vi "Poll iRobot and Accelerometer.vi"(6 "accel smoothing (0-1)":dbl=0.1, 8 "error in":errorcluster, 11 "UART port in":T10) -> (0 "error out":errorcluster, 1 "Acceleration (g)":T1 {"z axis (g)" format="%.3f"; "y axis (g)" format="%.3f"; "x axis (g)" format="%.3f"}, 2 "iRobot SensorGroup6":T2={"Bumps + Wheel Drops"={"Wheeldrop Caster"=FALSE, "Wheeldrop Left"=FALSE, "Wheeldrop Right"=FALSE, "Bump Left"=FALSE, "Bump Right"=FALSE}, "Wall"=FALSE, "Cliff Left"=FALSE, "Cliff Front Left"=FALSE, "Cliff Front Right"=FALSE, "Cliff Right"=FALSE, "Virtual Wall"=FALSE, "Low-Side Driver + Wheel Overcurrent"={"Low-Side Driver 0"=FALSE, "Low-Side Driver 1"=FALSE, "Low-Side Driver 2"=FALSE, "Left Wheel"=FALSE, "Right Wheel"=FALSE}, "Infrared"=255, "Buttons"={"Advance"=FALSE, "Play"=FALSE}, "Distance (mm)"=0, "Angle (deg)"=0, "Charging State"=enum."Not Charging", "Voltage (mV)"=0, "Current (mA)"=0, "Battery Temperature (deg C)"=0, "Battery Charge (mAh)"=0, "Battery Capacity (mAh)"=0, "Wall Signal (0-4095)"=0, "Cliff Left Signal (0-4095)"=0, "Cliff Front Left Signal (0-4095)"=0, "Cliff Front Right Signal (0-4095)"=0, "Cliff Right Signal (0-4095)"=0, "Cargo Bay Digital Inputs"={"Digital Input 0"=FALSE, "Digital Input 1"=FALSE, "Digital Input 2"=FALSE, "Digital Input 3"=FALSE, "Device Detect"=FALSE}, "Cargo Bay Analog Signal (0-1023)"=0, "Charging Sources Available"={"Internal Charger"=FALSE, "Home Base"=FALSE}, "OI Mode"=enum."Off", "Song Number"=0, "Song Playing"=FALSE, "Number of Stream Packets"=0, "Requested Velocity (mm/s)"=0, "Requested Radius (mm)"=0, "Requested Right Wheel Velocity (mm/s)"=0, "Requested Left Wheel Velocity (mm/s)"=0} {"Infrared" format="%02x"}, 3 "UART port out":T10, 5 "net angle (deg)":i32, 7 "net distance (mm)":i32)   [LabVIEW 2015]
uses:
  iRobot/Advanced/UART/iRobot UART Port Type.ctl
  iRobot/Sensor/Sensor Group 6.ctl
  iRobot/Sensor/Bumps + Wheel Drops.ctl
  iRobot/Sensor/Low-Side Driver + Wheel Overcurrent.ctl
  iRobot/Sensor/Buttons.ctl
  iRobot/Sensor/Charging State.ctl
  iRobot/Sensor/Cargo Bay Digital Inputs.ctl
  iRobot/Sensor/Charging Sources Available.ctl
  iRobot/Sensor/OI Mode.ctl
  Accelerometer.ctl
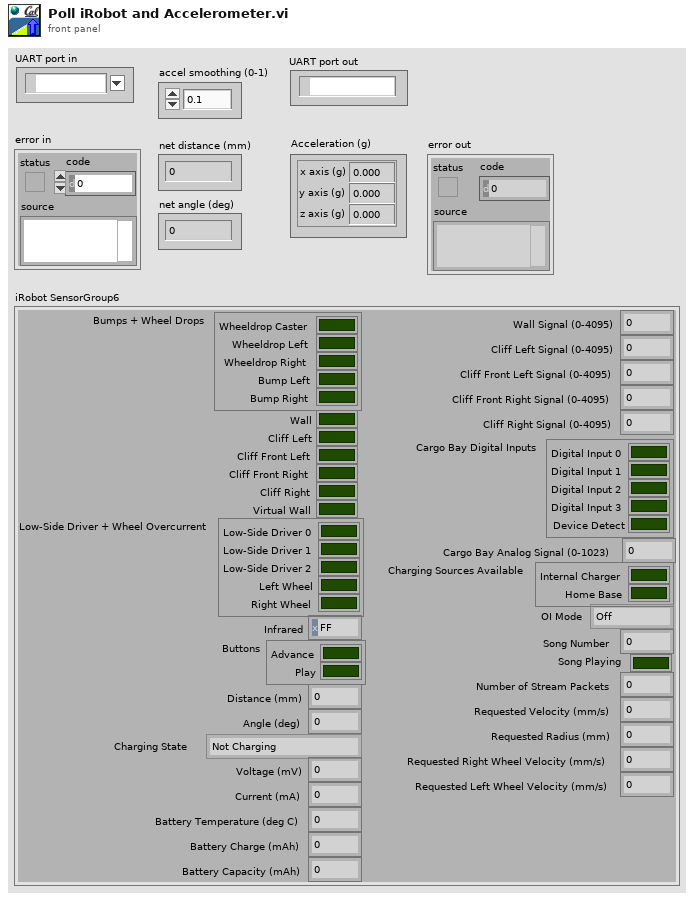
[diagram p1: front panel]
types:
  T1 = typedef "Accelerometer.ctl" = cluster{"x axis (g)":dbl, "y axis (g)":dbl, "z axis (g)":dbl}
  T2 = typedef "Sensor Group 6.ctl" = cluster{"Bumps + Wheel Drops":T3, "Wall":bool, "Cliff Left":bool, "Cliff Front Left":bool, "Cliff Front Right":bool, "Cliff Right":bool, "Virtual Wall":bool, "Low-Side Driver + Wheel Overcurrent":T4, "Infrared":u8, "Buttons":T5, "Distance (mm)":i32, "Angle (deg)":i32, "Charging State":T6, "Voltage (mV)":u16, "Current (mA)":i16, "Battery Temperature (deg C)":i8, "Battery Charge (mAh)":u16, "Battery Capacity (mAh)":u16, "Wall Signal (0-4095)":u16, "Cliff Left Signal (0-4095)":u16, "Cliff Front Left Signal (0-4095)":u16, "Cliff Front Right Signal (0-4095)":u16, "Cliff Right Signal (0-4095)":u16, "Cargo Bay Digital Inputs":T7, "Cargo Bay Analog Signal (0-1023)":u16, "Charging Sources Available":T8, "OI Mode":T9, "Song Number":u8, "Song Playing":bool, "Number of Stream Packets":u8, "Requested Velocity (mm/s)":i16, "Requested Radius (mm)":i16, "Requested Right Wheel Velocity (mm/s)":i16, "Requested Left Wheel Velocity (mm/s)":i16}
  T3 = typedef "Bumps + Wheel Drops.ctl" = cluster{"Wheeldrop Caster":bool, "Wheeldrop Left":bool, "Wheeldrop Right":bool, "Bump Left":bool, "Bump Right":bool}
  T4 = typedef "Low-Side Driver + Wheel Overcurrent.ctl" = cluster{"Low-Side Driver 0":bool, "Low-Side Driver 1":bool, "Low-Side Driver 2":bool, "Left Wheel":bool, "Right Wheel":bool}
  T5 = typedef "Buttons.ctl" = cluster{"Advance":bool, "Play":bool}
  T6 = typedef "Charging State.ctl" = enum16{"Not Charging", "Reconditioning Charging", "Full Charging", "Trickle Charging", "Waiting", "Charging Fault Condition"}
  T7 = typedef "Cargo Bay Digital Inputs.ctl" = cluster{"Digital Input 0":bool, "Digital Input 1":bool, "Digital Input 2":bool, "Digital Input 3":bool, "Device Detect":bool}
  T8 = typedef "Charging Sources Available.ctl" = cluster{"Internal Charger":bool, "Home Base":bool}
  T9 = typedef "OI Mode.ctl" = enum16{"Off", "Passive", "Safe", "Full"}
  T10 = typedef "iRobot UART Port Type.ctl" = refnum<visa-resource-name>
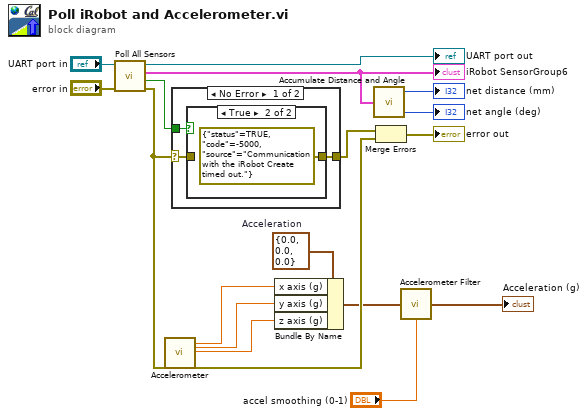
[diagram p0: block diagram]
diagram:
  w9 = T1 {"x axis (g)"=0.0, "y axis (g)"=0.0, "z axis (g)"=0.0}  # Acceleration
  n1 = call "Poll All Sensors.vi"("error in"="error in", "UART port in"="UART port in") -> ("error out"=w8:errorcluster, "Timed Out?"=w12:bool, "iRobot Sensors"=w18:T2, "UART port out"=→"UART port out":T10)  [unwired: 6 in]
  "iRobot SensorGroup6" <- w18
  n2 = call "Accelerometer"("error in (no error)"=w8) -> ("X-Axis"=w6:dbl, "Y-Axis"=w5:dbl, "Z-Axis"=w4:dbl, "error out"=w7:errorcluster)  [unwired: 23 in]
  n3 = case shown="No Error" w8 {
    selector: w8 -> [w19 w24]
    tunnel: w12 -> [w21 _]
    tunnel: [w20 w24] -> w10
    frame No Error {
      n4 = case shown="True" w21 {
        tunnel: [w22 errorcluster {"status"=TRUE, "code"=-5000, "source"="Communication with the iRobot Create timed out."} ("error constant")] -> w20
        tunnel: w19 -> [w22 _]
        frame False {
        }
        frame True {
        }
      }
    }
    frame Error {
    }
  }
  n5 = Bundle By Name(cluster=w9, "x axis (g)"=w6, "y axis (g)"=w5, "z axis (g)"=w4) -> (w3:T1)
  n6 = call "Accumulate Distance and Angle.vi"("iRobot SensorGroup6"=w18) -> ("net angle (mm)"=→"net angle (deg)":i32, "net distance (mm)"=→"net distance (mm)":i32)  [unwired: 3 in]
  n7 = Merge Errors(w10, w7) -> (→"error out":errorcluster)
  n8 = call "Accelerometer Filter.vi"("smoothing factor (0-1)"="accel smoothing (0-1)", "accelerometer (g)"=w3) -> ("filtered accelerometer (g)"=→"Acceleration (g)":T1)  [unwired: 2 in]
